vi "Read AI Array.vi"(8 "error in (no error)":errorcluster, 11 "FPGA in":refnum<class "FPGA.lvclass">) -> (0 "error out":errorcluster, 1 "AI Scaled Array":dbl[](array[numeric]), 2 "AI RAW Array":dbl[](array[numeric]), 3 "FPGA out":refnum<class "FPGA.lvclass">)   [LabVIEW 2019, in "FPGA.lvclass"]
uses:
  FPGA.lvclass
  FPGA.lvclass/FPGA.ctl
  <vilib>/Utility/error.llb/Error Cluster From Error Code.vi
  <vilib>/rvi/errors/niLvFpgaAdjustHostInterfaceError.vi
  <vilib>/rvi/interface/nirviReadWriteControl/nirviReadWriteControl.xnode
  FPGA VI Reference.ctl
  NiFpgaLv.dll
  <vilib>/rvi/interface/Simulation/niFpgaSimulationCallBeginRW.vi
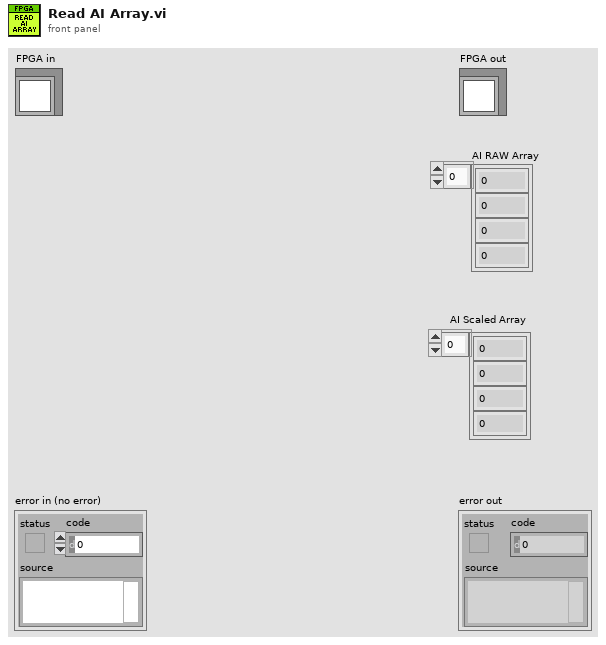
[diagram p1: front panel]
types:
  T1 = typedef "FPGA.lvclass/FPGA VI Reference.ctl" = refnum<k20>
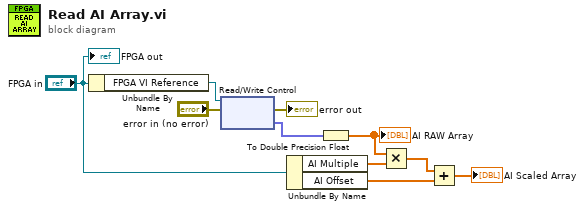
[diagram p0: block diagram]
diagram:
  n1 = Unbundle By Name("FPGA in") -> ("FPGA VI Reference"=w10:T1)
  n2 = xnode "Read/Write Control"("FPGA VI Reference In"=w10, "error in"="error in (no error)") -> ("error out"=→"error out":errorcluster, "AIs"=w8:fxp<+/-,21,-4>[])  [unwired: 1 out]
  n3 = Unbundle By Name("FPGA in") -> ("AI Multiple"=w2:dbl[], "AI Offset"=w1:dbl[])
  n4 = To Double Precision Float(number=w8) -> (double precision float=w6:dbl[])
  "AI RAW Array" <- w6
  n5 = Multiply(x=w6, y=w2) -> (x*y=w5:dbl[])
  n6 = Add(x=w5, y=w1) -> (x+y=→"AI Scaled Array":dbl[])
  "FPGA out" <- "FPGA in"
